vi "rvhr - Get Image Folder Info.vi"(6 "Local Data in":T1, 8 "error in (no error)":errorcluster, 11 "selected path":path) -> (0 "error out":errorcluster, 2 "Time Stamp":timestamp, 4 "Local Data out":T1)   [LabVIEW 2024]
uses:
  Controls/RVHR - Local Data.ctl
  Controls/Test Cluster.ctl
  Controls/Excluded Information.ctl
  Controls/Language.ctl
  Controls/Device_Type.ctl
  <vilib>/Utility/miscctls.llb/LVRectTypeDef.ctl
  <vilib>/Utility/miscctls.llb/LVBoundsTypeDef.ctl
  <vilib>/Analysis/NI_AALBase.lvlib
  <vilib>/Analysis/1siggen.llb/Ramp Pattern by Samples.vi
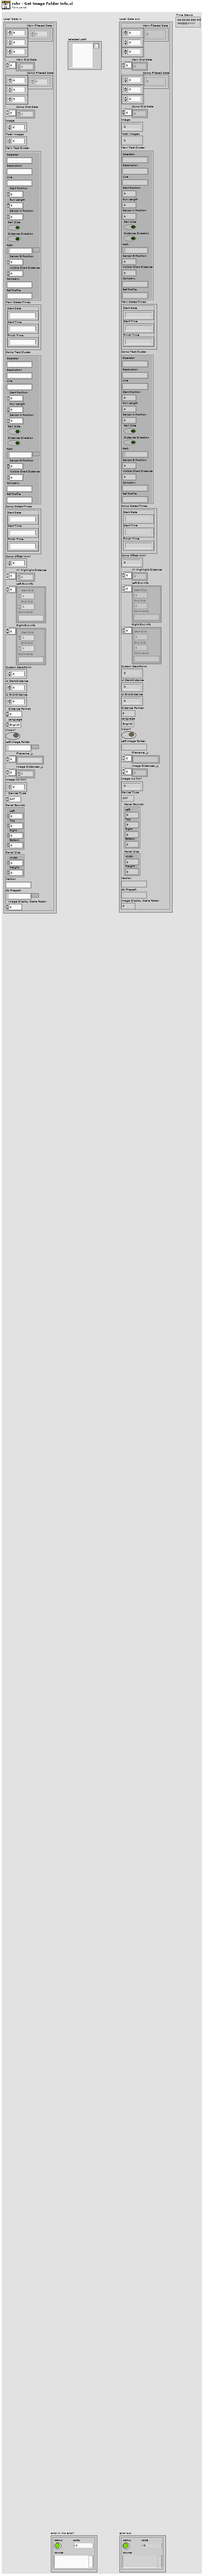
[diagram p1: front panel]
types:
  T1 = typedef "RVHR - Local Data.ctl" = cluster{"Main Filtered Data":dbl[][][], "Main Dist Data":dbl[], "Comp Filtered Data":dbl[][][], "Comp Dist Data":dbl[], "Image":u16, "Total Images":u16, "Main Test Cluster":T2, "Main Dates-Times":cluster{"Start Date":string, "Start Time":string, "Finish Time":string}, "Comp Test Cluster":T2, "Comp Dates-Times":cluster{"Start Date":string, "Start Time":string, "Finish Time":string}, "Comp Offset (mm)":i64, "XY Highlight Distance":dbl[], "Left Exc Info":T3[], "Right Exc Info":T3[], "Custom Start-Point":dbl, "UI Start-Distance":dbl, "UI End-Distance":dbl, "Distance Format":u8, "Language":T4, "Vision?":bool, "Left Image Folder":path, "Filename _L":string[], "Image Distances _L":dbl[], "Image Inc (km)":dbl, "Device Type":T5, "Panel Bounds":T6, "Panel Size":T7, "Version":string, "db Filepath":path, "Image Display Scale Factor":dbl}
  T2 = typedef "Test Cluster.ctl" = cluster{"Operator":string, "Description":string, "Line":string, "Start Position":dbl, "Run Length":dbl, "Sensor A Position":dbl, "Rail Side":bool, "Distance Direction":bool, "Path":path, "Sensor B Position":dbl, "Visible Chart Distance":dbl, "Company":string, "Ref Profile":string}
  T3 = typedef "Excluded Information.ctl" = cluster{"Start Dist":dbl, "End Dist":dbl, "Comments":string}
  T4 = typedef "Language.ctl" = enum16{"English", "Chinese", "German"}
  T5 = typedef "Device_Type.ctl" = enum16{"CAT", "Bi-CAT", "YRCA", "RCA", "RV-HR", "TV-HR"}
  T6 = typedef "LVRectTypeDef.ctl" = cluster{"Left":i16, "Top":i16, "Right":i16, "Bottom":i16}
  T7 = typedef "LVBoundsTypeDef.ctl" = cluster{"Width":u32, "Height":u32}
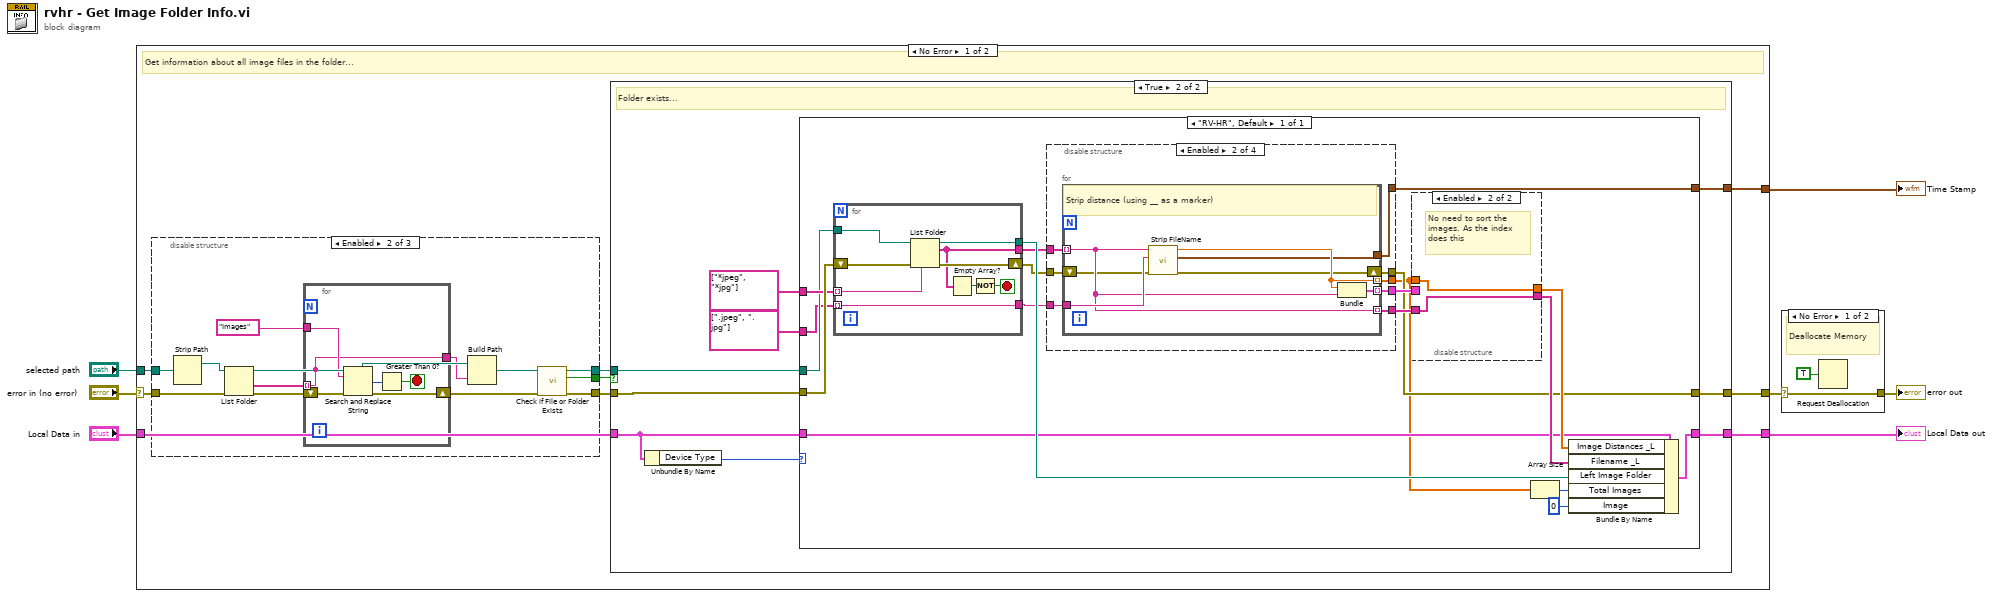
[diagram p0: block diagram]
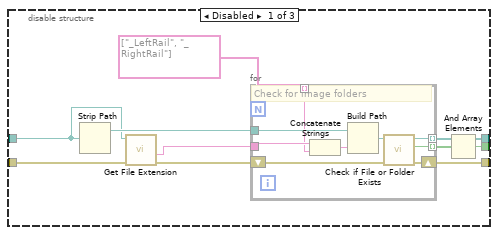
[diagram p3: hidden frame]
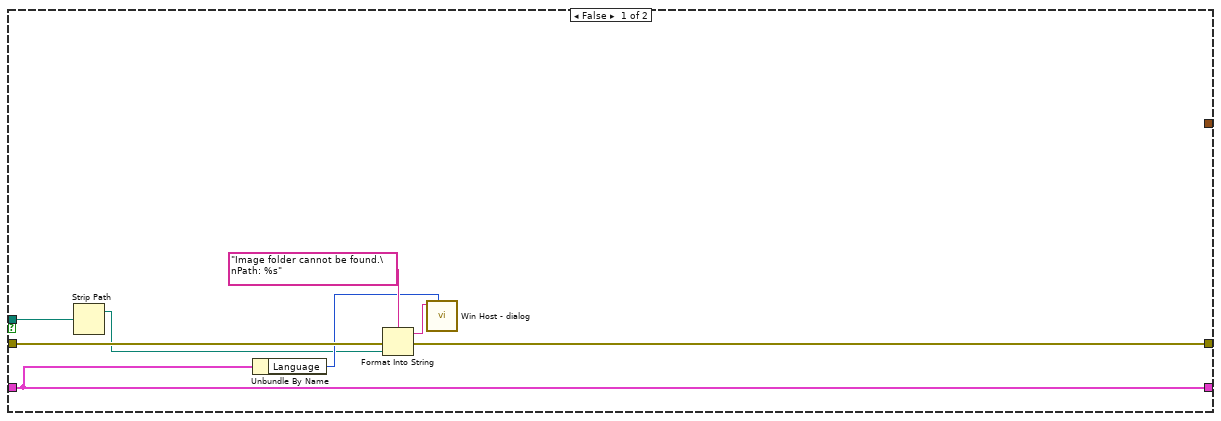
[diagram p5: hidden frame]
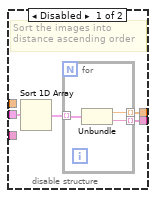
[diagram p6: hidden frame]
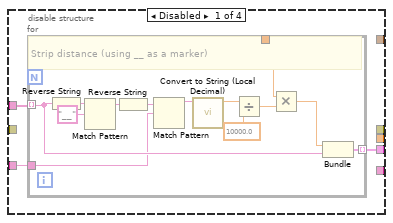
[diagram p7: hidden frame]
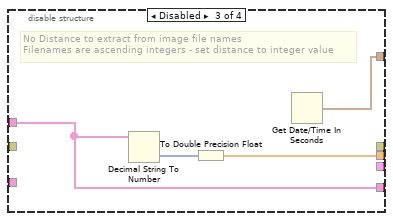
[diagram p8: hidden frame]
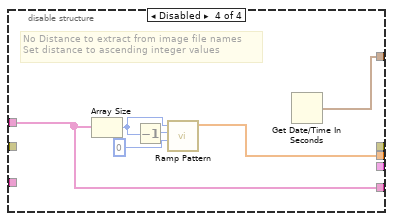
[diagram p9: hidden frame]
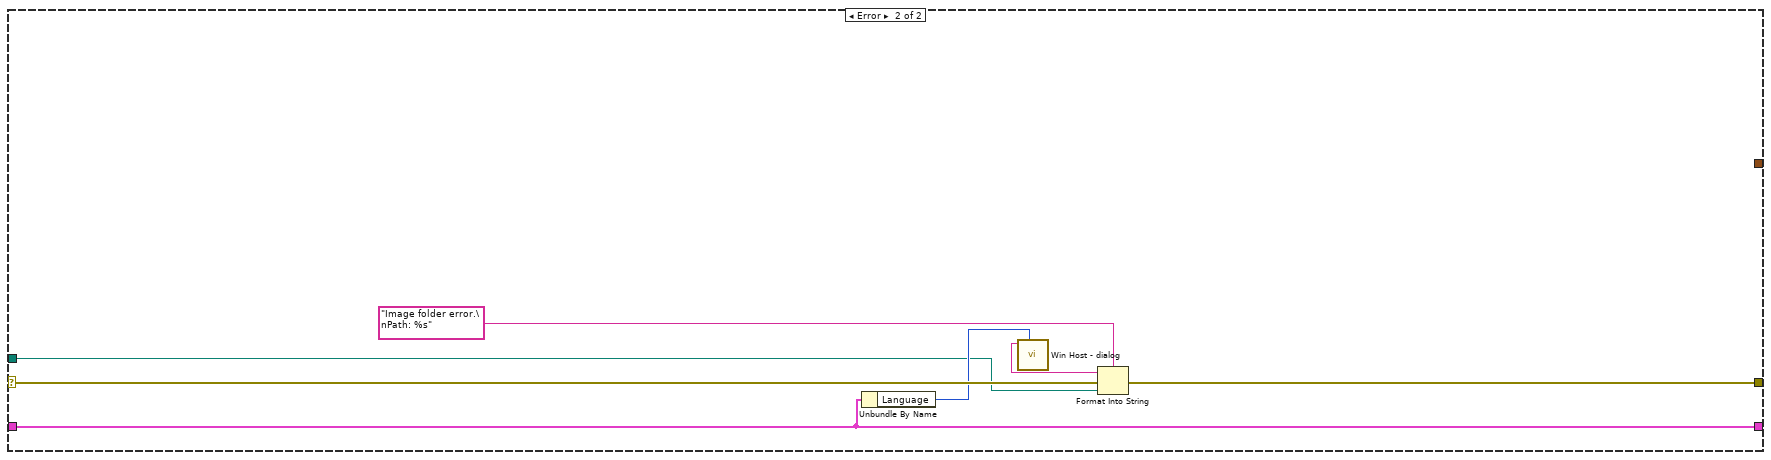
[diagram p10: hidden frame]
diagram:
  n1 = case shown="No Error" "error in (no error)" {
    selector: "error in (no error)" -> [w16 w155]
    tunnel: "selected path" -> [w9 w151]
    tunnel: "Local Data in" -> [w14 w153]
    tunnel: [w13 w153] -> w4
    tunnel: [w12 w154] -> w2
    tunnel: [w8 _] -> w3
    frame No Error {
      # "Get information about all image files in the folder..."
      n2 = disable-structure shown="Enabled" {
        disable-tunnel: w16 -> [w26 w45 _]
        disable-tunnel: [w25 w48 _] -> w15
        disable-tunnel: [w21 w47 _] -> w11
        disable-tunnel: [w20 w36 _] -> w10
        disable-tunnel: w9 -> [w18 w46 _]
        frame Disabled {
          n3 = Strip Path(path=w18) -> (stripped path=w23:path)  [unwired: 1 out]
          n4 = call <vilib>:"Get File Extension.vi"("error in (no error)"=w26, "file"=w18) -> ("error out"=w19:errorcluster, "filename without extension"=w17:string)  [unwired: 5 in, 3 out]
          n5 = for {
            tunnel: [w33] -> w24 mode=indexing
            shift-right: [w34] -> w25
            shift-left: w19 -> [w35]
            tunnel: w23 -> [w31]
            tunnel: w17 -> [w30]
            tunnel: string[] ["_LeftRail", "_RightRail"] -> [w28] mode=indexing
            tunnel: [w27] -> w21 mode=indexing
            # "Check for image folders"
            n6 = Concatenate Strings(w30, w28) -> (w29:string)
            n7 = Build Path(base path=w31, name or relative path=w29) -> (appended path=w32:path)
            n8 = call <vilib>:"Check if File or Folder Exists.vi"("error in (no error)"=w35, "path"=w32) -> ("error out"=w34:errorcluster, "file or folder exists?"=w33:bool, "dup path"=w27:path)  [unwired: 7 in]
          }
          n9 = And Array Elements(Boolean array=w24) -> (logical AND=w20:bool)
        }
        frame Enabled {
          n10 = Strip Path(path=w46) -> (stripped path=w44:path)  [unwired: 1 out]
          n11 = List Folder(path=w44, error in=w45) -> (path out=w43:path, folder names=w40:string[], error out=w41:errorcluster)  [unwired: 2 in, 1 out]
          n12 = for {
            tunnel: "Images" -> [w53]
            shift-right: [w51] -> w38
            shift-left: w41 -> [w54]
            tunnel: w40 -> [w49] mode=indexing
            tunnel: [w49] -> w37
            stop <- w50 stop-if-true
            n13 = Search and Replace String(input string=w49, search string=w53, error in=w54) -> (number of replacements=w52:i32, error out=w51:errorcluster)  [unwired: 5 in, 2 out]
            n14 = Greater Than 0?(x=w52) -> (x > 0?=w50:bool)
          }
          n15 = Build Path(base path=w43, name or relative path=w37) -> (appended path=w39:path)
          n16 = call <vilib>:"Check if File or Folder Exists.vi"("error in (no error)"=w38, "path"=w39) -> ("error out"=w48:errorcluster, "file or folder exists?"=w36:bool, "dup path"=w47:path)  [unwired: 7 in]
        }
        frame Disabled {
        }
      }
      n17 = case shown="True" w10 {
        tunnel: w15 -> [w61 w71]
        tunnel: w11 -> [w56 w70]
        tunnel: w14 -> [w58 w67]
        tunnel: [w58 w69] -> w13
        tunnel: [w60 w68] -> w12
        tunnel: [_ w63] -> w8
        frame False {
          n18 = Strip Path(path=w56) -> (stripped path=w55:path)  [unwired: 1 out]
          n19 = Unbundle By Name(w58) -> ("Language"=w57:T4)
          n20 = Format Into String(format string="Image folder cannot be found.\nPath: %s" ("Message"), error in=w61, w55) -> (resulting string=w59:string, error out=w60:errorcluster)  [unwired: 1 in]
          n21 = call "Win Host - dialog.vi"("Language"=w57, "Message"=w59) -> ()  [unwired: 8 in, 2 out]
        }
        frame True {
          # "Folder exists..."
          n22 = Unbundle By Name(w67) -> ("Device Type"=w66:T5)
          n23 = case shown="\"RV-HR\", Default" w66 {
            tunnel: w71 -> [w84]
            tunnel: w70 -> [w81]
            tunnel: w67 -> [w83]
            tunnel: [w89] -> w69
            tunnel: [w76] -> w68
            tunnel: string[] ["*jpeg", "*jpg"] -> [w82]
            tunnel: string[] [".jpeg", ".jpg"] -> [w79]
            tunnel: [w75] -> w63
            frame "RV-HR", Default {
              n24 = for {
                tunnel: [w150] -> w90
                tunnel: w81 -> [w142]
                tunnel: [w146] -> w85
                shift-right: [w148] -> w77
                shift-left: w84 -> [w149]
                tunnel: w82 -> [w147] mode=indexing
                tunnel: w79 -> [w143] mode=indexing
                tunnel: [w143] -> w80
                stop <- w144 stop-if-true
                n25 = List Folder(path=w142, pattern=w147, error in=w149) -> (path out=w150:path, filenames=w146:string[], error out=w148:errorcluster)  [unwired: 1 in, 1 out]
                n26 = Empty Array?(array=w146) -> (empty?=w145:bool)
                n27 = Not(x=w145) -> (.not. x?=w144:bool)
              }
              n28 = disable-structure shown="Enabled" {
                disable-tunnel: [w103 w124 _ _] -> w86
                disable-tunnel: w85 -> [w102 w123 w132 w137]
                disable-tunnel: w80 -> [w100 w122 _ _]
                disable-tunnel: [_ w121 w134 w136] -> w72
                disable-tunnel: [_ w120 w132 w137] -> w78
                disable-tunnel: w77 -> [_ w118 _ _]
                disable-tunnel: [_ w119 _ _] -> w76
                disable-tunnel: [_ w117 w133 w141] -> w75
                frame Disabled {
                  n29 = for {
                    tunnel: w102 -> [w113] mode=indexing
                    tunnel: [w112] -> w103 mode=indexing
                    tunnel: [w106] -> w101
                    tunnel: w100 -> [w104]
                    # "Strip distance (using __ as a marker)"
                    n30 = Reverse String(1:w113) -> (0:w115:string)
                    n31 = Match Pattern(string=w115, regular expression="__") -> (before substring=w114:string)  [unwired: 1 in, 3 out]
                    n32 = Reverse String(1:w114) -> (0:w111:string)
                    n33 = Match Pattern(string=w111, regular expression=w104) -> (before substring=w110:string)  [unwired: 1 in, 3 out]
                    n34 = call "Convert to String (Local Decimal).vi"("Distance (String)"=w110) -> ("Distance (DBL)"=w109:dbl)  [unwired: 10 in]
                    n35 = Divide(x=w109, y=10000.0) -> (x/y=w107:dbl)
                    n36 = Multiply(x=w106, y=w107) -> (x*y=w105:dbl)
                    n37 = Bundle(w105, w113) -> (w112:cluster{dbl, string})  [unwired: 1 in]
                  }
                }
                frame Enabled {
                  n38 = for {
                    tunnel: w123 -> [w128] mode=indexing
                    tunnel: [w131] -> w124 mode=indexing
                    tunnel: w122 -> [w130]
                    tunnel: [w129] -> w121 mode=indexing
                    tunnel: [w128] -> w120 mode=indexing
                    shift-right: [w126] -> w119
                    shift-left: w118 -> [w127]
                    tunnel: [w125] -> w117
                    # "Strip distance (using __ as a marker)"
                    n39 = call "Strip FileName.vi"("error in"=w127, "File Type"=w130, "Filename"=w128) -> ("error out"=w126:errorcluster, "Time Stamp"=w125:timestamp, "Distance (DBL)"=w129:dbl)  [unwired: 6 in]
                    n40 = Bundle("Distance (DBL)"=w129, w128) -> (w131:cluster{"Distance (DBL)":dbl, string})  [unwired: 1 in]
                  }
                }
                frame Disabled {
                  # "No Distance to extract from image file names\nFilenames are ascending integers - set distance to integer value"
                  n41 = Decimal String To Number(string=w132) -> (number=w135:i32[])  [unwired: 2 in, 1 out]
                  n42 = To Double Precision Float(number=w135) -> (double precision float=w134:dbl[])
                  n43 = Get Date/Time In Seconds() -> (seconds since 1Jan1904=w133:timestamp)
                }
                frame Disabled {
                  # "No Distance to extract from image file names\nSet distance to ascending integer values"
                  n44 = Array Size(array=w137) -> (size(s)=w139:i32)
                  n45 = Decrement(x=w139) -> (x-1=w140:i32)
                  n46 = call-poly <vilib>:"Ramp Pattern.vi"("start"=0 ("size(s)"), "end"=w140, "samples"=w139) -> ("Ramp Pattern"=w136:dbl[])  [unwired: 7 in, 1 out]
                  n47 = Get Date/Time In Seconds() -> (seconds since 1Jan1904=w141:timestamp)
                }
              }
              n48 = disable-structure shown="Enabled" {
                disable-tunnel: [w93 w99] -> w88
                disable-tunnel: [w92 w98] -> w87
                disable-tunnel: w86 -> [w91 _]
                disable-tunnel: w72 -> [_ w98]
                disable-tunnel: w78 -> [_ w99]
                frame Disabled {
                  # "Sort the images into\ndistance ascending order"
                  n49 = Sort 1D Array(array=w91) -> (sorted array=w94:cluster{"Distance (DBL)":dbl, string}[])
                  n50 = for {
                    tunnel: w94 -> [w97] mode=indexing
                    tunnel: [w96] -> w92 mode=indexing
                    tunnel: [w95] -> w93 mode=indexing
                    n51 = Unbundle(w97) -> ("Distance (DBL)"=w96:dbl, w95:string)
                  }
                }
                frame Enabled {
                  # "No need to sort the\nimages. As the index\ndoes this"
                }
              }
              n52 = Array Size(array=w72) -> (size(s)=w73:i32)
              n53 = Bundle By Name(cluster=w83, "Image Distances _L"=w87, "Filename _L"=w88, "Left Image Folder"=w90, "Total Images"=w73, "Image"=u8 0) -> (w89:T1)
            }
          }
        }
      }
    }
    frame Error {
      n54 = Unbundle By Name(w153) -> ("Language"=w152:T4)
      n55 = Format Into String(format string="Image folder error.\nPath: %s" ("Message"), error in=w155, w151) -> (resulting string=w156:string, error out=w154:errorcluster)  [unwired: 1 in]
      n56 = call "Win Host - dialog.vi"("Language"=w152, "Message"=w156) -> ()  [unwired: 8 in, 2 out]
    }
  }
  "Local Data out" <- w4
  "Time Stamp" <- w3
  n57 = case shown="No Error" w2 {
    selector: w2 -> [w158 w160]
    tunnel: [w158 w160] -> w1
    frame No Error {
      # "Deallocate Memory"
      n58 = Request Deallocation(TRUE ("flag")) -> ()
    }
    frame Error {
    }
  }
  "error out" <- w1
